vi "Userevent driver.vi"(0 "Event data":cluster{"Stop":bool}, 11 "Error in":errorcluster, 13 "Mode":T1) -> (4 "Data type":refnum<user-event>, 15 "Error out":errorcluster)   [LabVIEW 2020, in "Producer&Consumer - Washing Machine.lvlib"]
uses:
  Producer&Consumer - Washing Machine.lvlib
  Userevent driver mode.ctl
  Userevent datatype.ctl
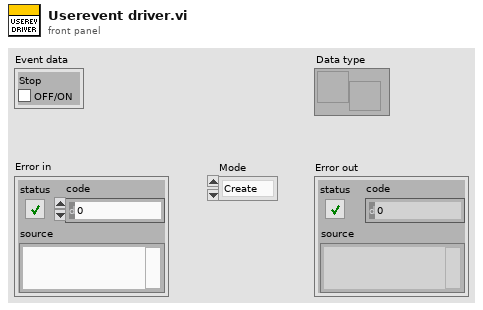
[diagram p1: front panel]
types:
  T1 = typedef "Producer&Consumer - Washing Machine.lvlib/Userevent driver mode.ctl" = enum16{"Create", "Generate", "Read", "Destroy"}
  T2 = typedef "Producer&Consumer - Washing Machine.lvlib/Userevent datatype.ctl" = cluster{"Stop":bool}
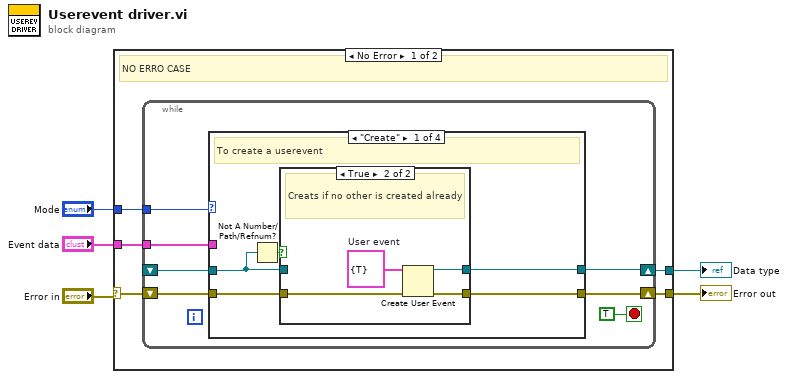
[diagram p0: block diagram]
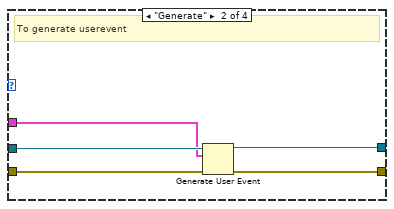
[diagram p3: hidden frame]
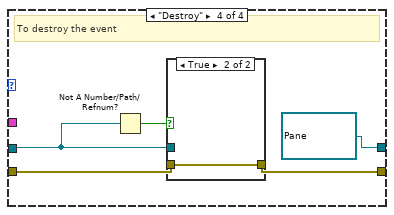
[diagram p5: hidden frame]
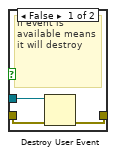
[diagram p6: hidden frame]
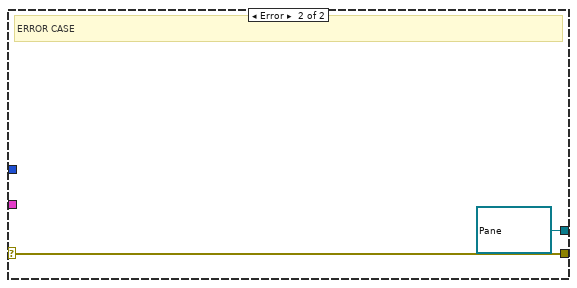
[diagram p7: hidden frame]
diagram:
  n1 = case shown="No Error" "Error in" {
    selector: "Error in" -> [w8 w46]
    tunnel: "Mode" -> [w10 _]
    tunnel: [w9 w46] -> w3
    tunnel: "Event data" -> [w7 _]
    tunnel: [w6 refnum<user-event> refnum ("Data type")] -> w1
    frame No Error {
      # "NO ERRO CASE"
      n2 = while {
        tunnel: w10 -> [w17]
        shift-right: [w16] -> w9
        shift-left: w8 -> [w15]
        shift-right: [w13] -> w6
        shift-left: _ -> [w12]
        tunnel: w7 -> [w11]
        stop <- TRUE stop-if-true
        n3 = case shown="\"Create\"" w17 {
          tunnel: [w21 w32 w35 w39] -> w16
          tunnel: w15 -> [w22 w33 w35 w40]
          tunnel: [w20 w30 w34 refnum<user-event> refnum ("Data type")] -> w13
          tunnel: w12 -> [w18 w31 w34 w38]
          tunnel: w11 -> [_ w29 _ _]
          frame "Create" {
            # "To create a userevent"
            n4 = Not A Number/Path/Refnum?(number/path/refnum=w18) -> (NaN/Path/Refnum?=w19:bool)
            n5 = case shown="True" w19 {
              tunnel: w22 -> [w23 w28]
              tunnel: [w23 w27] -> w21
              tunnel: [w24 w25] -> w20
              tunnel: w18 -> [w24 _]
              frame False {
              }
              frame True {
                w26 = T2 {"Stop"=TRUE}  # User event
                # "Creats if no other is created already"
                n6 = Create User Event(user event datatype=w26, error in=w28) -> (user event=w25:refnum<user-event>, error out=w27:errorcluster)
              }
            }
          }
          frame "Generate" {
            # "To generate userevent"
            n7 = Generate User Event(user event=w31, event data cluster=w29, error in=w33) -> (user event out=w30:refnum<user-event>, error out=w32:errorcluster)  [unwired: 1 in]
          }
          frame "Read" {
            # "To read the event"
          }
          frame "Destroy" {
            # "To destroy the event"
            n8 = Not A Number/Path/Refnum?(number/path/refnum=w38) -> (NaN/Path/Refnum?=w37:bool)
            n9 = case shown="True" w37 {
              tunnel: w40 -> [w43 w44]
              tunnel: [w42 w44] -> w39
              tunnel: w38 -> [w41 _]
              frame False {
                # "If event is available means it will destroy"
                n10 = Destroy User Event(user event=w41, error in=w43) -> (error out=w42:errorcluster)
              }
              frame True {
              }
            }
          }
        }
      }
    }
    frame Error {
      # "ERROR CASE"
    }
  }
  "Error out" <- w3
  "Data type" <- w1
